vi "General Polynomial Fit Coefficients (LS).vi"(0 "Y":dbl[](array[numeric]), 1 "polynomial order":i32=2, 2 "Coefficient Constraint":cluster{"order":i32, "coefficient":dbl}[](array[cluster]), 5 "X":dbl[](array[numeric]), 7 "Weight":dbl[](array[numeric]), 13 "algorithm":T1 items=["SVD", "Givens", "Givens2", "Householder", "LU Decomposition", "Cholesky", "SVD for Rank Deficient H"]) -> (4 "Polynomial Coefficients":dbl[](array[numeric]), 15 "error":i32)   [LabVIEW 2018, in "NI_AALPro.lvlib"]
uses:
  <vilib>/Analysis/NI_AALPro.lvlib
  <vilib>/Analysis/6fits.llb/General Linear Fit Algorithm.ctl
  <resource>/lvanlys.dll
panel:
  # "LS General Polynomial Fit Coefficients"
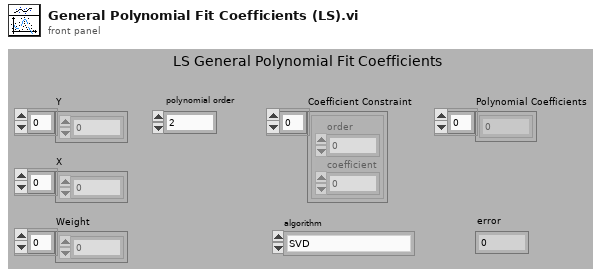
[diagram p1: front panel]
types:
  T1 = typedef "NI_AALPro.lvlib/General Linear Fit Algorithm.ctl" = u16
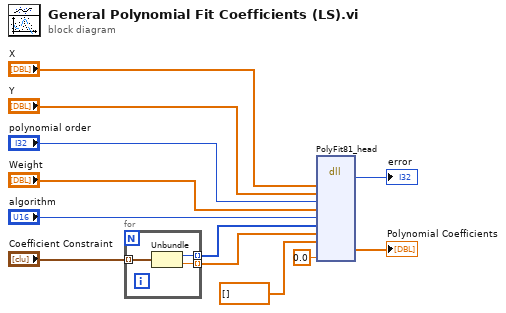
[diagram p0: block diagram]
diagram:
  n1 = for {
    tunnel: "Coefficient Constraint" -> [w15] mode=indexing
    tunnel: [w14] -> w4 mode=indexing
    tunnel: [w13] -> w5 mode=indexing
    n2 = Unbundle(w15) -> ("order"=w14:i32, "coefficient"=w13:dbl)
  }
  n3 = dll-call lib="C:/Program Files (x86)/National Instruments/LabVIEW 2018/resource/lvanlys.*" fn="PolyFit81_head"("xH"="X", "yH"="Y", "Order"="polynomial order", "weightH"="Weight", "algorithm"="algorithm", "specOrderH"=w4, "specCoefH"=w5, "BestFitH"=dbl[] [], "mse"=0.0) -> ("return type"=→"error":i32, "CoefH"=→"Polynomial Coefficients":dbl[])  [unwired: 11 in, 4 out]
